vi "read_logger_event.vi"(11 "ev":T1) -> (2 "ev":T1, 3 "return":i16)   [LabVIEW 2011]
uses:
  canopen_dll_master.dll
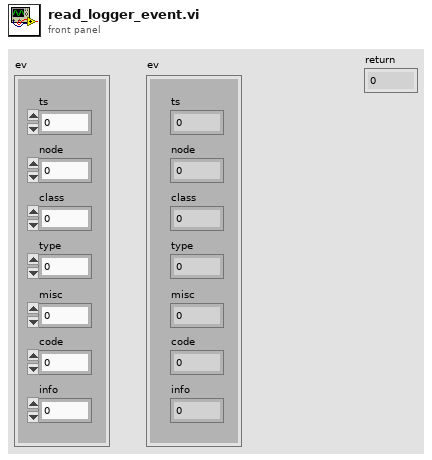
[diagram p1: front panel]
types:
  T1 = cluster{"ts":i64, "node":u8, "class":u8, "type":u8, "misc":u8, "code":i16, "info":i32}
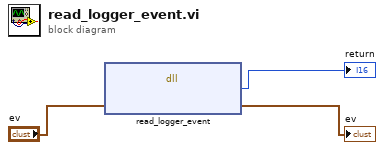
[diagram p0: block diagram]
diagram:
  n1 = dll-call lib="canopen_dll_master.dll" fn="read_logger_event"("ev"="ev") -> ("return type"=→"return":i16, "ev"=→"ev":T1)  [unwired: 3 in, 2 out]
